vi "Build Tree Data Type.vi"(4 "Show IDs (True)":bool=TRUE, 6 "Indent":i32, 7 "Tag Blacklist":i8[](array[numeric]), 8 "error in (no error)":errorcluster, 9 "Items":T1(array[cluster]), 10 "Child IDs":string[](array[string]), 11 "ILinked List in":refnum<class "ILinked List.lvclass">) -> (0 "error out":errorcluster, 1 "Items Out":T1(array[cluster]), 3 "ILinked List out":refnum<class "ILinked List.lvclass">)   [LabVIEW 2019, in "Linked Lists.lvlib" / "ILinked List.lvclass"]
uses:
  <vilib>/gpm_packages/@cs/linked-list/Source/Linked List/ILinkedList/ILinked List.lvclass
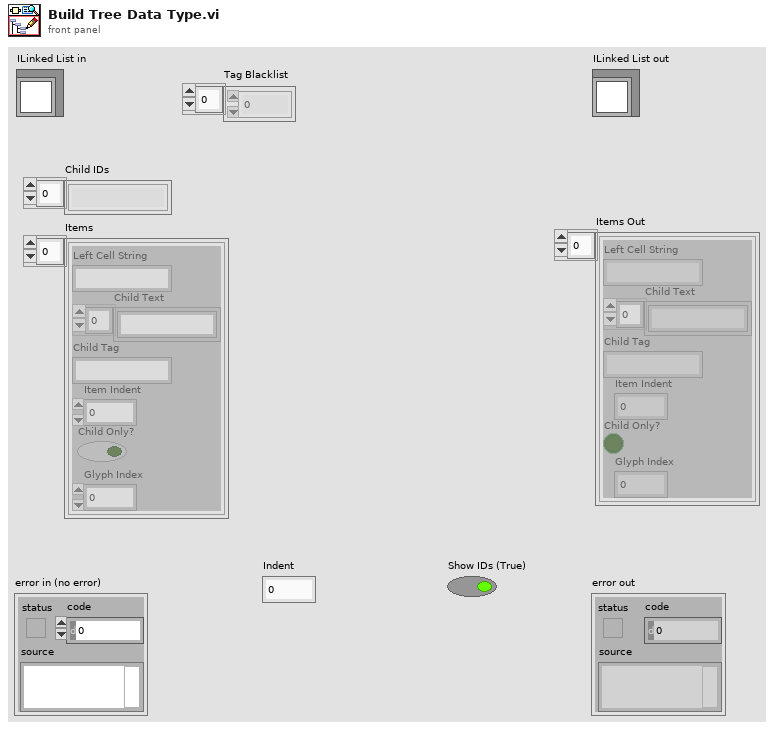
[diagram p1: front panel]
types:
  T1 = cluster{"Left Cell String":string, "Child Text":string[], "Child Tag":string, "Item Indent":i32, "Child Only?":bool, "Glyph Index":i32}[]
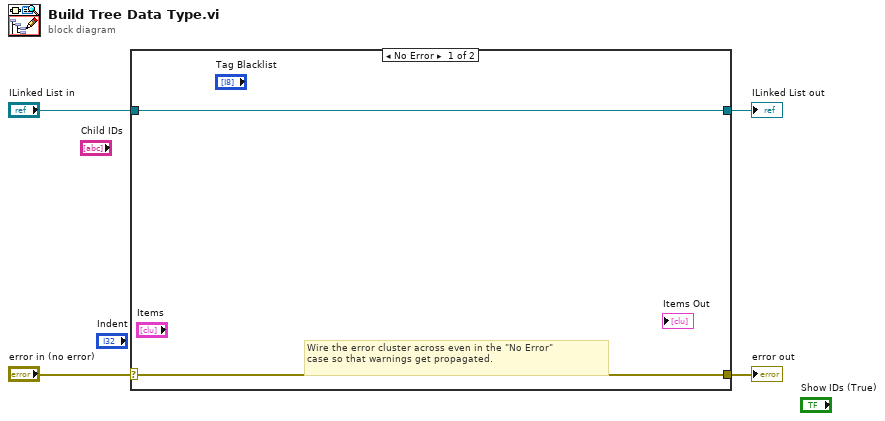
[diagram p0: block diagram]
diagram:
  n1 = case shown="No Error" "error in (no error)" {
    selector: "error in (no error)" -> [w5 w8]
    tunnel: [w5 w8] -> w3
    tunnel: [w6 w7] -> w1
    tunnel: "ILinked List in" -> [w6 w7]
    frame No Error {
      # "Wire the error cluster across even in the \"No Error\"\ncase so that warnings get propagated."
    }
    frame Error {
    }
  }
  "error out" <- w3
  "ILinked List out" <- w1
